vi "magazine_globals.vi"() -> ()   [LabVIEW 2020]
panel:
  out "Eject Command":bool
  out "Outtake Command":bool
  out "Intake Command":bool
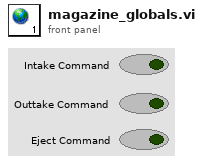
[diagram p1: front panel]
diagram:
